vi "TIFF Register CODEC.vi"(8 "error in (no error)":errorcluster, 9 "para2":cluster{}, 10 "para1":cluster{}, 11 "para0":cluster{}) -> (0 "error out":errorcluster, 3 "function return":u32)   [LabVIEW 2018]
doc: "LIBTIFF_DLL_IMPEXP TIFFCodec* TIFFRegisterCODEC(uint16, const char*, TIFFInitMethod);\nextern TIFFCodec* TIFFRegisterCODEC(uint16, const char*, TIFFInitMethod);"
uses:
  libtiff3.dll
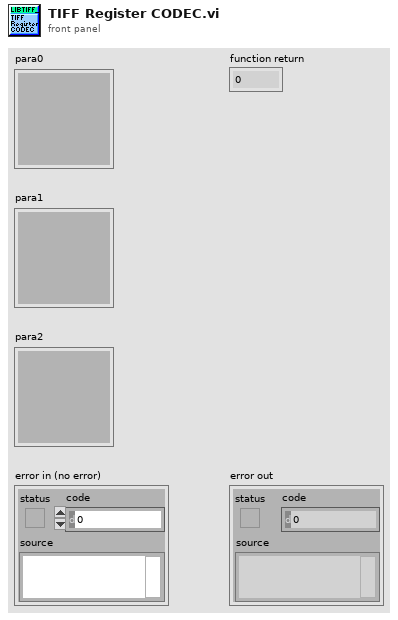
[diagram p1: front panel]
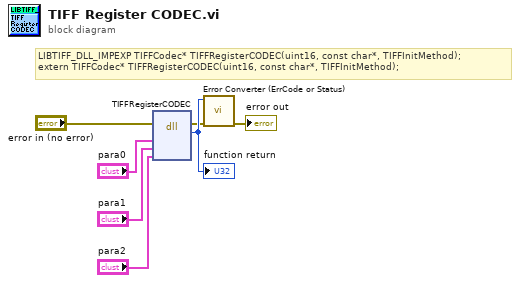
[diagram p0: block diagram]
diagram:
  # "LIBTIFF_DLL_IMPEXP\tTIFFCodec* TIFFRegisterCODEC(uint16, const char*, TIFFInitMethod);\nextern\tTIFFCodec* TIFFRegisterCODEC(uint16, const char*, TIFFInitMethod);"
  n1 = dll-call lib="C:/Users/johan/Downloads/LabVIEW software/LabVIEW software/IX-81 Software/lib/tiff/LibTiffLabview/libtiff3.*" fn="TIFFRegisterCODEC"(error in="error in (no error)", "para0"="para0", "para1"="para1", "para2"="para2") -> (error out=w2:errorcluster, w7:u32)  [unwired: 5 in, 1 out]
  "function return" <- w7
  n2 = call "Error Converter (ErrCode or Status).vi"("error in (no error)"=w2, "error code"=w7) -> ("error out"=→"error out":errorcluster)  [unwired: 9 in]
